vi "DOTNET - Set JPEG Quality.vi"(7 "Quality":u8=100, 11 "error in (no error)":errorcluster) -> (4 "ImageCodecInfo":refnum<k24>, 8 "EncoderParameters":refnum<k24>, 15 "error out":errorcluster)   [LabVIEW 2016]
uses:
  System.Drawing
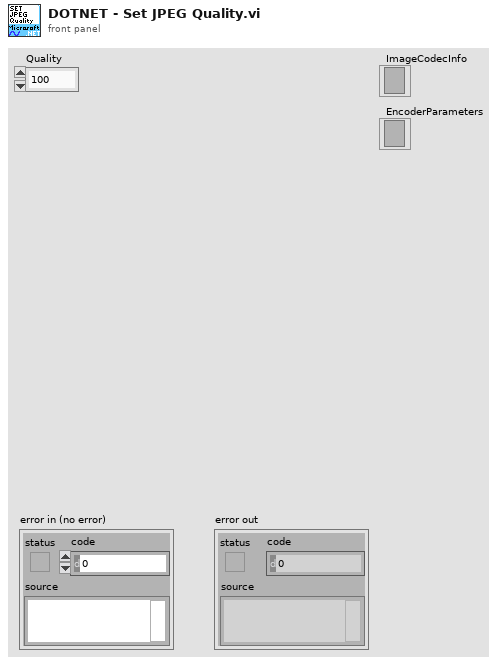
[diagram p1: front panel]
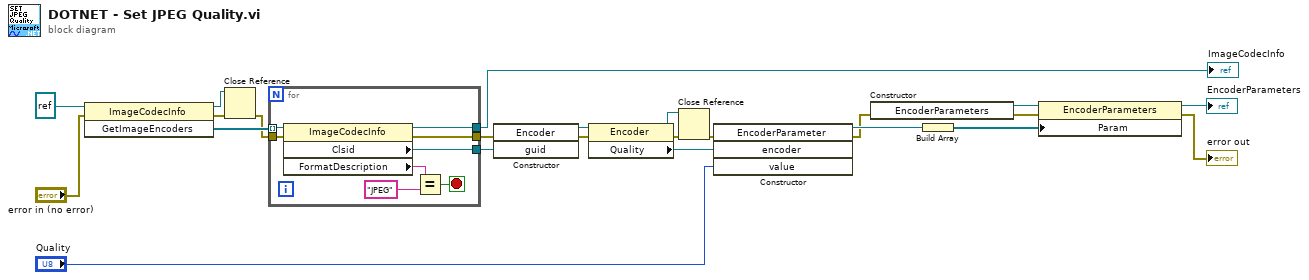
[diagram p0: block diagram]
diagram:
  n1 = invoke class="ImageCodecInfo" method="GetImageEncoders"(reference=refnum<k24> refnum ("encoder"), error in="error in (no error)") -> (reference out=w1:refnum<k24>, error out=w15:errorcluster, "GetImageEncoders"=w22:refnum<k24>[])  [unwired: 1 in]
  n2 = Close Reference(reference=w1, error in (no error)=w15) -> (error out=w2:errorcluster)
  n3 = for {
    tunnel: w22 -> [w31] mode=indexing
    tunnel: w2 -> [w27]
    tunnel: [w26] -> w14
    tunnel: [w25] -> w13
    tunnel: [w24] -> w3
    stop <- w28 stop-if-true
    n4 = property class="ImageCodecInfo"(reference=w31, error in=w27) -> (reference out=w24:refnum<k24>, error out=w25:errorcluster, "Clsid"=w26:refnum<k24>, "FormatDescription"=w30:string)
    n5 = Equal?(x=w30, y="JPEG" ("element")) -> (x = y?=w28:bool)
  }
  "ImageCodecInfo" <- w3
  n6 = constructor class="Encoder"(error in=w13, "guid"=w14) -> (reference out=w21:refnum<k24>, error out=w12:errorcluster)  [unwired: 2 in, 2 out]
  n7 = property class="Encoder"(reference=w21, error in=w12) -> (reference out=w4:refnum<k24>, error out=w11:errorcluster, "Quality"=w6:refnum<k24>)
  n8 = Close Reference(reference=w4, error in (no error)=w11) -> (error out=w5:errorcluster)
  n9 = constructor class="EncoderParameter"(error in=w5, "encoder"=w6, "value"="Quality") -> (reference out=w17:refnum<k24>, error out=w10:errorcluster)  [unwired: 2 in, 3 out]
  n10 = constructor class="EncoderParameters"(error in=w10) -> (reference out=w20:refnum<k24>, error out=w19:errorcluster)  [unwired: 2 in, 1 out]
  n11 = Build Array(w17) -> (w16:refnum<k24>[])
  n12 = property class="EncoderParameters"(reference=w20, error in=w19, "Param"=w16) -> (reference out=→"EncoderParameters":refnum<k24>, error out=→"error out":errorcluster)
